vi "Task1_UTC_2_UTCSEC.vi"() -> (3 "UTCSec":dbl, 11 "current time":timestamp)   [LabVIEW 2024]
panel:
  out "date/time string":string
  in  "stop":bool
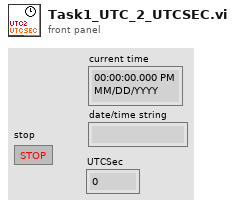
[diagram p1: front panel]
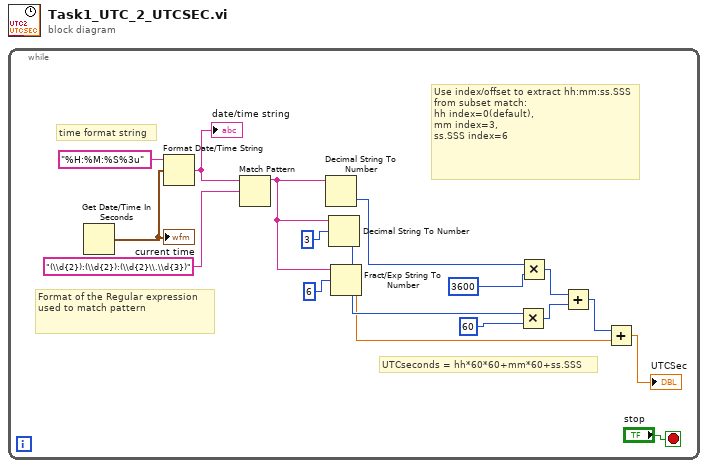
[diagram p0: block diagram]
diagram:
  n1 = while {
    stop <- "stop" stop-if-true
    # "UTCseconds = hh*60*60+mm*60+ss.SSS"
    # "Use index/offset to extract hh:mm:ss.SSS from subset match: \nhh index=0(default), \nmm index=3,\nss.SSS index=6"
    # "time format string"
    # "Format of the Regular expression used to match pattern"
    n2 = Get Date/Time In Seconds() -> (seconds since 1Jan1904=w15:timestamp)
    "current time" <- w15
    n3 = Format Date/Time String(time format string (%c)="%H:%M:%S%3u", seconds (now)=w15) -> (date/time string=w14:string)  [unwired: 1 in]
    "date/time string" <- w14
    n4 = Match Pattern(string=w14, regular expression="(\\d{2}):(\\d{2}):(\\d{2}\\.\\d{3})") -> (before substring=w11:string)  [unwired: 1 in, 3 out]
    n5 = Decimal String To Number(string=w11) -> (number=w9:i32)  [unwired: 2 in, 1 out]
    n6 = Decimal String To Number(string=w11, offset=3) -> (number=w7:i32)  [unwired: 1 in, 1 out]
    n7 = Fract/Exp String To Number(string=w11, offset=6) -> (number=w3:dbl)  [unwired: 2 in, 1 out]
    n8 = Multiply(x=w7, y=60) -> (x*y=w4:i32)
    n9 = Multiply(x=w9, y=3600) -> (x*y=w5:i32)
    n10 = Add(x=w5, y=w4) -> (x+y=w2:i32)
    n11 = Add(x=w2, y=w3) -> (x+y=→"UTCSec":dbl)
  }
